vi "Reg0Write UnitTest Python.vi"() -> ()   [LabVIEW 2018]
uses:
  Command/RFFE Command.lvclass
  Downloads/MIPI RFFE API/Controls/RFFE Commands Type Def.ctl
  Downloads/MIPI RFFE API/Controls/Write Data Strict Type Def.ctl
  RegReadExt/RFFE RegReadExt Command.lvclass
  C:/Users/semoore/Projects/mipi-rffe-labview-oop/api/RFFE Command.lvclass
panel:
  out "x = y? 3":bool
  out "x = y? 2":bool
  out "logical AND 2":bool
  out "x = y?":bool
  out "logical AND":bool
  out "error in (no error) 2":errorcluster
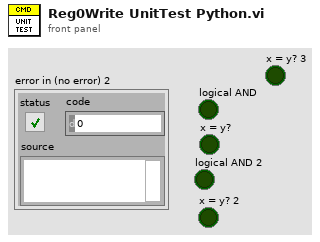
[diagram p1: front panel]
types:
  T1 = typedef "Write Data Strict Type Def.ctl" = cluster{"slave address":u8, "register address":u16, "register data (write)":u8[], "byte count":u8}
  T2 = typedef "RFFE Commands Type Def.ctl" = enum16{"Reg0Write", "RegWrite", "RegRead", "RegReadHR", "RegWriteExt", "RegReadExt", "RegReadExtHR", "RegWriteExtLong", "RegReadExtLong", "RegReadExtLongHR"}
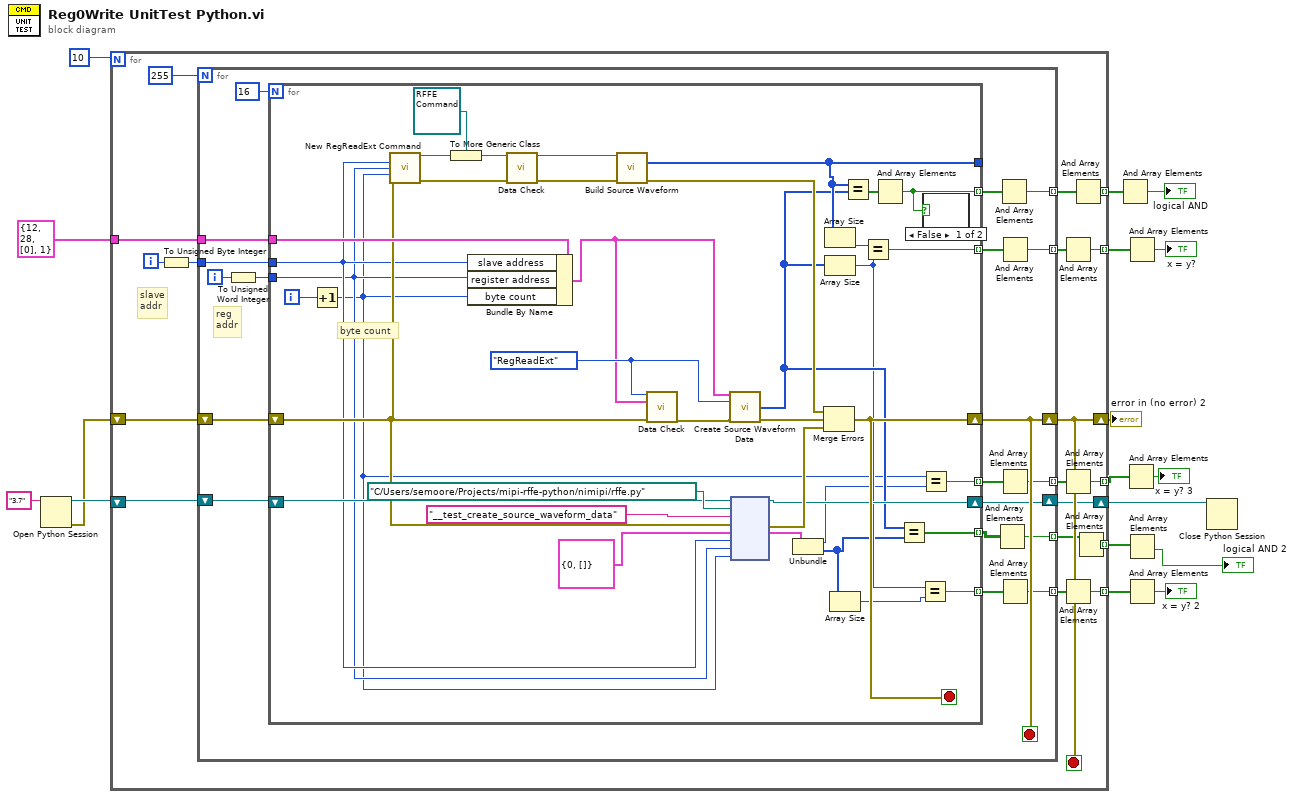
[diagram p0: block diagram]
diagram:
  n1 = Open Python Session(python version="3.7" ("Python version")) -> (session out=w11:refnum<k35>, error out=w9:errorcluster)  [unwired: 2 in]
  n2 = for {
    N: 10 -> [_]
    tunnel: T1 {"slave address"=12, "register address"=28, "register data (write)"=[0], "byte count"=1} ("Register Data") -> [w34]
    shift-right: [w31] -> w15
    shift-left: w9 -> [w35]
    tunnel: [w29] -> w14 mode=indexing
    shift-right: [w27] -> w10
    shift-left: w11 -> [w28]
    tunnel: [w25] -> w8 mode=indexing
    tunnel: [w23] -> w6 mode=indexing
    tunnel: [w22] -> w3 mode=indexing
    tunnel: [w18] -> w2 mode=indexing
    i -> [w33]
    stop <- w31 stop-if-true
    # "slave\naddr"
    n3 = To Unsigned Byte Integer(number=w33) -> (unsigned 8bit integer=w20:u8)
    n4 = for {
      N: 255 -> [_]
      tunnel: w34 -> [w53]
      tunnel: w20 -> [w50]
      shift-right: [w49] -> w31
      shift-left: w35 -> [w54]
      tunnel: [w47] -> w30 mode=indexing
      shift-right: [w45] -> w27
      shift-left: w28 -> [w46]
      tunnel: [w43] -> w26 mode=indexing
      tunnel: [w41] -> w24 mode=indexing
      tunnel: [w40] -> w21 mode=indexing
      tunnel: [w36] -> w19 mode=indexing
      i -> [w51]
      stop <- w49 stop-if-true
      # "reg\naddr"
      n5 = To Unsigned Word Integer(number=w51) -> (unsigned 16bit integer=w38:u16)
      n6 = for {
        N: 16 -> [_]
        tunnel: w53 -> [w90]
        tunnel: [w78] -> _
        tunnel: w38 -> [w58]
        tunnel: w50 -> [w59]
        shift-right: [w81] -> w49
        shift-left: w54 -> [w72]
        tunnel: [w76] -> w48 mode=indexing
        shift-right: [w69] -> w45
        shift-left: w46 -> [w70]
        tunnel: [w66] -> w44 mode=indexing
        tunnel: [w65] -> w42 mode=indexing
        tunnel: [w64] -> w39 mode=indexing
        tunnel: [w55] -> w37 mode=indexing
        i -> [w60]
        stop <- w81 stop-if-true
        w92 = RFFE_Commands_Type_Def."RegReadExt" ("RFFE command")
        # "byte count"
        n7 = Increment(x=w60) -> (x+1=w56:i32)
        n8 = call "New RegReadExt Command.vi"("Slave Address"=w59, "Register Address"=w58, "Byte Count"=w56, "error in (no error)"=w72) -> ("RFFE RegReadExt Command out"=w85:refnum<class "RFFE RegReadExt Command.lvclass">, "error out"=w87:errorcluster)  [unwired: 10 in]
        n9 = To More Generic Class(target class=refnum<class "RFFE Command.lvclass"> refnum ("RFFE Commands.lvlib:RFFE Command.lvclass"), reference=w85) -> (generic class reference=w86:refnum<class "RFFE Command.lvclass">)
        n10 = Bundle By Name(cluster=w90, "slave address"=w59, "register address"=w58, "byte count"=w56) -> (w89:T1)
        n11 = call-dynamic "Data Check.vi"("RFFE Command in"=w86, "error in (no error)"=w87) -> ("RFFE Command out"=w84:refnum<class "RFFE Command.lvclass">, "error out"=w88:errorcluster)  [unwired: 12 in]
        n12 = call-dynamic "Build Source Waveform.vi"("RFFE Command in"=w84, "error in (no error)"=w88) -> ("Source Waveform"=w78:u32[], "error out"=w80:errorcluster)  [unwired: 11 in, 1 out]
        n13 = call "Data Check.vi"("RFFE command"=w92, "Register Data"=w89, "error in"=w72) -> ("error out"=w91:errorcluster)  [unwired: 12 in]
        n14 = call "Create Source Waveform Data.vi"("Register Data"=w89, "RFFE command"=w92, "error in"=w91) -> ("RFFEWrite source waveform data array"=w67:u32[], "error out"=w82:errorcluster)  [unwired: 10 in, 1 out]
        n15 = node(w70, path "C:/Users/semoore/Projects/mipi-rffe-python/nimipi/rffe.py" ("module path"), "__test_create_source_waveform_data" ("function name"), w72, cluster{i32, u32[]} {0, []}, w59, w58, w56) -> (w69:refnum<k35>, w71:errorcluster, w68:cluster{i32, u32[]})  [unwired: 3 in, 2 out]
        n16 = Unbundle(w68) -> (w57:i32, w62:u32[])
        n17 = Merge Errors(w80, w82, w71) -> (w81:errorcluster)
        n18 = Array Size(array=w78) -> (size(s)=w77:i32)
        n19 = Array Size(array=w67) -> (size(s)=w63:i32)
        n20 = Array Size(array=w62) -> (size(s)=w61:i32)
        n21 = Equal?(x=w78, y=w67) -> (x = y?=w79:bool[])
        n22 = Equal?(x=w77, y=w63) -> (x = y?=w65:bool)
        n23 = And Array Elements(Boolean array=w79) -> (logical AND=w76:bool)
        n24 = Equal?(x=w67, y=w62) -> (x = y?=w66:bool[])
        n25 = Equal?(x=w63, y=w61) -> (x = y?=w64:bool)
        n26 = Equal?(x=w56, y=w57) -> (x = y?=w55:bool)
        n27 = case shown="False" w76 {
          frame False {
          }
          frame True {
          }
        }
      }
      n28 = And Array Elements(Boolean array=w44) -> (logical AND=w43:bool)
      n29 = And Array Elements(Boolean array=w48) -> (logical AND=w47:bool)
      n30 = And Array Elements(Boolean array=w42) -> (logical AND=w41:bool)
      n31 = And Array Elements(Boolean array=w37) -> (logical AND=w36:bool)
      n32 = And Array Elements(Boolean array=w39) -> (logical AND=w40:bool)
    }
    n33 = And Array Elements(Boolean array=w24) -> (logical AND=w23:bool)
    n34 = And Array Elements(Boolean array=w19) -> (logical AND=w18:bool)
    n35 = And Array Elements(Boolean array=w21) -> (logical AND=w22:bool)
    n36 = And Array Elements(Boolean array=w30) -> (logical AND=w29:bool)
    n37 = And Array Elements(Boolean array=w26) -> (logical AND=w25:bool)
  }
  "error in (no error) 2" <- w15
  n38 = And Array Elements(Boolean array=w14) -> (logical AND=→"logical AND":bool)
  n39 = And Array Elements(Boolean array=w2) -> (logical AND=→"x = y? 3":bool)
  n40 = And Array Elements(Boolean array=w6) -> (logical AND=→"x = y?":bool)
  n41 = And Array Elements(Boolean array=w8) -> (logical AND=→"logical AND 2":bool)
  n42 = And Array Elements(Boolean array=w3) -> (logical AND=→"x = y? 2":bool)
  n43 = Close Python Session(session in=w10) -> ()  [unwired: 1 in, 1 out]
